vi "http parse header string.vi"(11 "raw string":string) -> (0 "no field name":bool, 1 "no crlf":bool, 2 "header field data":string, 3 "header field name":string, 5 "continuation":bool)   [LabVIEW 2013, in "http headers.lvlib"]
uses:
  http headers.lvlib
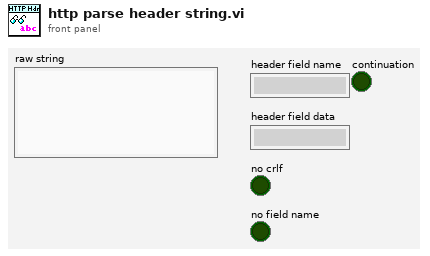
[diagram p1: front panel]
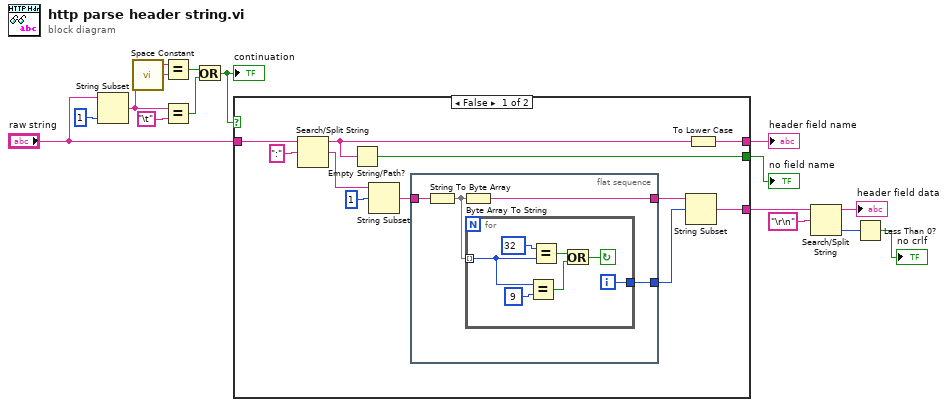
[diagram p0: block diagram]
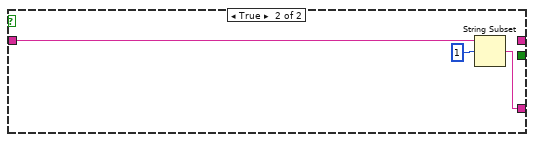
[diagram p2: hidden frame]
diagram:
  n1 = String Subset(string="raw string", length (rest)=1 ("length (rest)")) -> (substring=w9:string)  [unwired: 1 in]
  n2 = call <vilib>:"Space Constant.vi"() -> ("String"=w8:string)
  n3 = Equal?(x=w9, y=w8) -> (x = y?=w12:bool)
  n4 = Equal?(x=w9, y="\t") -> (x = y?=w11:bool)
  n5 = Or(x=w12, y=w11) -> (x .or. y?=w6:bool)
  "continuation" <- w6
  n6 = case shown="False" w6 {
    tunnel: [w26 _] -> w15
    tunnel: "raw string" -> [w24 w40]
    tunnel: [w25 _] -> w10
    tunnel: [w17 w38] -> w5
    frame False {
      n7 = Search/Split String(string=w24, search string/char (-)=":" ("regular expression")) -> (substring before match=w22:string, match + rest of string=w20:string)  [unwired: 1 in, 1 out]
      n8 = Empty String/Path?(string/path=w22) -> (empty?=w26:bool)
      n9 = String Subset(string=w20, offset (0)=1) -> (substring=w19:string)  [unwired: 1 in]
      n10 = flat-sequence {
        tunnel: w19 -> [w30]
        tunnel: [w28] -> w16
        tunnel: [w29] -> w18
        frame #0 {
          n11 = String To Byte Array(string=w30) -> (unsigned byte array=w27:u8[])
          n12 = Byte Array To String(unsigned byte array=w27) -> (string=w28:string)
          n13 = for {
            tunnel: w27 -> [w37] mode=indexing
            tunnel: [w31] -> w29
            i -> [w31]
            stop <- w32 continue-if-true
            n14 = Equal?(x=w37, y=u8 9) -> (x = y?=w35:bool)
            n15 = Equal?(x=u8 32 ("y"), y=w37) -> (x = y?=w36:bool)
            n16 = Or(x=w36, y=w35) -> (x .or. y?=w32:bool)
          }
        }
      }
      n17 = String Subset(string=w16, offset (0)=w18) -> (substring=w17:string)  [unwired: 1 in]
      n18 = To Lower Case(string=w22) -> (all lower case string=w25:string)
    }
    frame True {
      n19 = String Subset(string=w40, offset (0)=1) -> (substring=w38:string)  [unwired: 1 in]
    }
  }
  "no field name" <- w15
  "header field name" <- w10
  n20 = Search/Split String(string=w5, search string/char (-)="\r\n" ("regular expression")) -> (substring before match=→"header field data":string, offset of match=w2:i32)  [unwired: 1 in, 1 out]
  n21 = Less Than 0?(x=w2) -> (x < 0?=→"no crlf":bool)
